vi "Untitled 3 (SubVI).vi"(10 "Multicolumn Listbox in":refnum<vi>, 11 "MulticolumnListbox in":refnum<vi>) -> ()   [LabVIEW 2020, in "History.lvlib"]
uses:
  History.lvlib
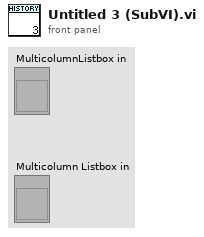
[diagram p1: front panel]
types:
  T1 = enum16{"open", "replace", "create", "open or create", "replace or create", "replace or create with confirmation"}
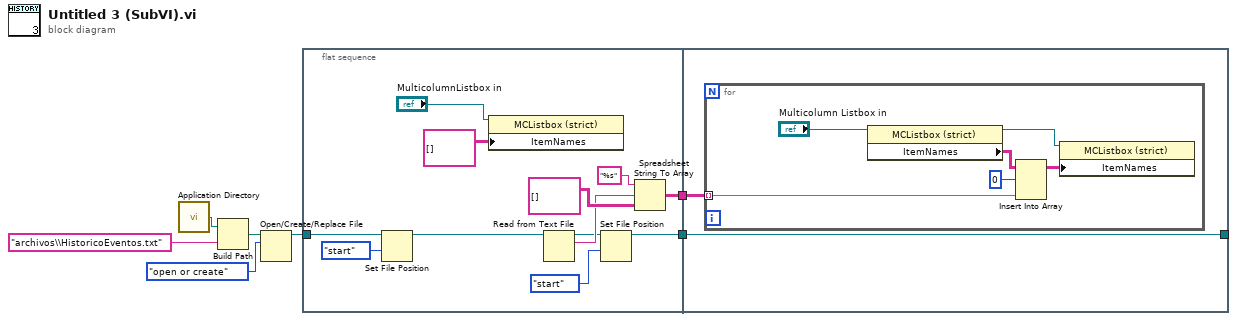
[diagram p0: block diagram]
diagram:
  n1 = call <vilib>:"Application Directory.vi"() -> ("Application Directory"=w1:path)
  n2 = Build Path(base path=w1, name or relative path="archivos\\HistoricoEventos.txt") -> (appended path=w3:path)
  n3 = Open/Create/Replace File(file path (use dialog)=w3, operation (0:open)=T1."open or create") -> (refnum out=w5:refnum<file>)  [unwired: 4 in, 2 out]
  n4 = flat-sequence {
    tunnel: w5 -> [w11]
    tunnel: [w15] -> w7
    tunnel: [w9] -> w6
    tunnel: w7 -> [w21]
    tunnel: [w20] -> _
    tunnel: w6 -> [w20]
    frame #0 {
      n5 = Set File Position(refnum=w11, from (0:start)=enum16{"start", "end", "current"}."start") -> (refnum out=w10:refnum<file>)  [unwired: 2 in, 1 out]
      n6 = property on="Property Node" class="MCListbox (strict)"(reference="MulticolumnListbox in", "ItemNames"=string[][] [] ("Array")) -> ()  [unwired: 1 in, 2 out]
      n7 = Read from Text File(file (use dialog)=w10) -> (refnum out=w14:refnum<file>, text=w17:string)  [unwired: 2 in, 3 out]
      n8 = Set File Position(refnum=w14, from (0:start)=enum16{"start", "end", "current"}."start") -> (refnum out=w9:refnum<file>)  [unwired: 2 in, 1 out]
      n9 = Spreadsheet String To Array(format string="%s", spreadsheet string=w17, array type (2D Dbl)=string[][] [] ("Array")) -> (array=w15:string[][])  [unwired: 1 in]
    }
    frame #1 {
      n10 = for {
        tunnel: w21 -> [w25] mode=indexing
        n11 = property on="Property Node" class="MCListbox (strict)"(reference="Multicolumn Listbox in") -> (reference out=w22:refnum<vi>, "ItemNames"=w27:string[][])  [unwired: 1 in, 1 out]
        n12 = Insert Into Array(array=w27, index (row)=0, new element=w25) -> (w26:string[][])  [unwired: 1 in]
        n13 = property on="Property Node" class="MCListbox (strict)"(reference=w22, "ItemNames"=w26) -> ()  [unwired: 1 in, 2 out]
      }
    }
  }
